vi "Run.vi"(8 "error in (no error)":errorcluster, 11 "Project in":refnum<class "Run VI.lvclass">) -> (0 "error out":errorcluster, 2 "Text":string, 3 "Project out":refnum<class "Run VI.lvclass">)   [LabVIEW 2014, in "Run VI.lvclass"]
uses:
  Run VI.lvclass
  Run VI.lvclass/Run VI.ctl
  Build Job/Build Job.lvclass/Build Job.ctl
  Build Job/Read Hostname.vi
  Build Job/Read Job Build Info.vi
  Build Job/Read Parameters.vi
  Build Job/Write Parameters.vi
  Build Job/Build Job.lvclass
  <vilib>/wsapi/NI_WebServices.lvlib
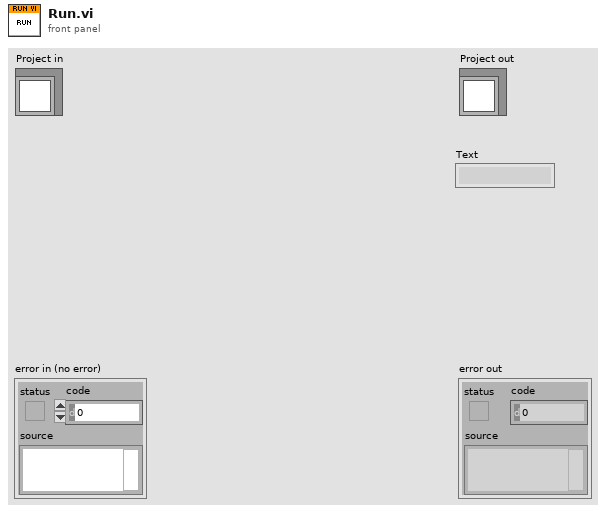
[diagram p1: front panel]
types:
  T1 = typedef "Run VI - STYP.ctl" = cluster{"Executor_Number":string, "VI_Path":string, "Wait_Until_Done":bool}
  T2 = typedef "Job Build Info - STYP.ctl" = cluster{"Build Name":string, "Description":string, "Notification":string, "Artifact Days":string, "Project Folder":string}
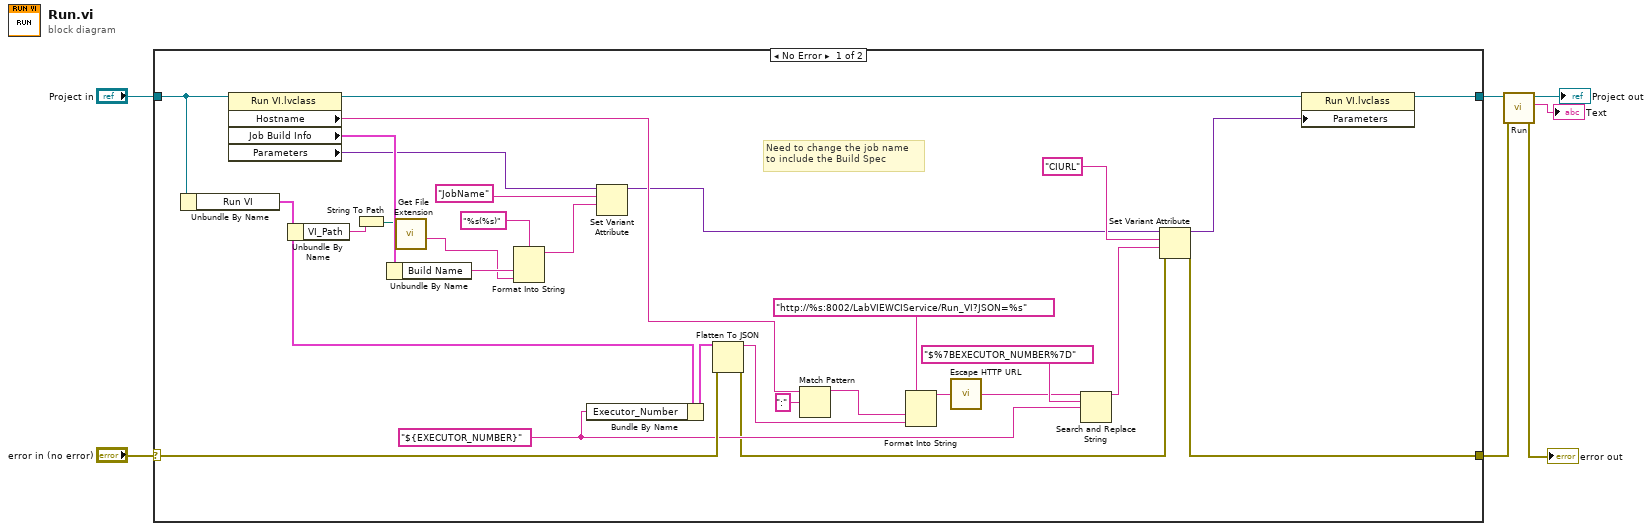
[diagram p0: block diagram]
diagram:
  n1 = case shown="No Error" "error in (no error)" {
    selector: "error in (no error)" -> [w36 w39]
    tunnel: [w18 w39] -> w2
    tunnel: [w37 w38] -> w1
    tunnel: "Project in" -> [w23 w38]
    frame No Error {
      w27 = "${EXECUTOR_NUMBER}" ("Executor_Number")
      # "Need to change the job name\nto include the Build Spec"
      n2 = Unbundle By Name(w23) -> ("Run VI"=w16:T1)
      n3 = property class="Run VI.lvclass"(reference=w23) -> (reference out=w22:refnum<class "Run VI.lvclass">, "Hostname"=w21:string, "Job Build Info"=w20:T2, "Parameters"=w12:variant)  [unwired: 1 in, 1 out]
      n4 = Unbundle By Name(w16) -> ("VI_Path"=w9:string)
      n5 = String To Path(string=w9) -> (path=w10:path)
      n6 = Unbundle By Name(w20) -> ("Build Name"=w14:string)
      n7 = call <vilib>:"Get File Extension.vi"("file"=w10) -> ("filename without extension"=w8:string)  [unwired: 7 in, 3 out]
      n8 = Format Into String(format string="%s(%s)", w14, w8) -> (resulting string=w13:string)  [unwired: 2 in, 1 out]
      n9 = Bundle By Name(cluster=w16, "Executor_Number"=w27) -> (w31:T1)
      n10 = Set Variant Attribute(Variant=w12, name="JobName" ("Name"), value=w13) -> (Variant out=w11:variant)  [unwired: 1 in, 2 out]
      n11 = Flatten To JSON(anything=w31, error in (no error)=w36) -> (JSON string=w32:string, 11:w19:errorcluster)  [unwired: 1 in]
      n12 = Match Pattern(string=w21, regular expression=":") -> (before substring=w33:string)  [unwired: 1 in, 3 out]
      n13 = Format Into String(format string="http://%s:8002/LabVIEWCIService/Run_VI?JSON=%s", w33, w32) -> (resulting string=w30:string)  [unwired: 2 in, 1 out]
      n14 = call <vilib>:"Escape HTTP URL.vi"("unescaped string in"=w30) -> ("escaped string out"=w28:string)
      n15 = Search and Replace String(input string=w28, search string="$%7BEXECUTOR_NUMBER%7D" ("replace string (\"\")"), replace string=w27) -> (result string=w25:string)  [unwired: 5 in, 3 out]
      n16 = Set Variant Attribute(Variant=w11, name="CIURL" ("Name"), value=w25, error in=w19) -> (Variant out=w24:variant, error out=w18:errorcluster)  [unwired: 1 out]
      n17 = property class="Run VI.lvclass"(reference=w22, "Parameters"=w24) -> (reference out=w37:refnum<class "Run VI.lvclass">)  [unwired: 1 in, 1 out]
    }
    frame Error {
    }
  }
  n18 = call-parent "Run.vi"("error in (no error)"=w2, "Project in"=w1) -> ("error out"=→"error out":errorcluster, "Text"=→"Text":string, "Project out"=→"Project out":refnum<class "Run VI.lvclass">)  [unwired: 7 in]
